vi "Product Page.vi"() -> (0 "Error Out":errorcluster)   [LabVIEW 2013, in "LVH-XBMC.lvlib"]
uses:
  vi.lib/LabVIEW Hacker/XBMC/LVH-XBMC.lvlib
  <vilib>/Platform/browser.llb/Open URL in Default Browser (string).vi
  <vilib>/LabVIEW Hacker/LVH-Toolbox/Common/LVH-Common.lvlib
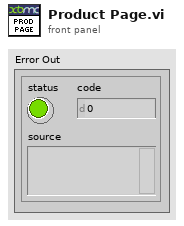
[diagram p1: front panel]
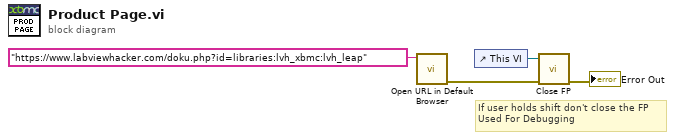
[diagram p0: block diagram]
diagram:
  # "If user holds shift don't close the FP\nUsed For Debugging"
  n1 = call-poly <vilib>:"Open URL in Default Browser.vi"("URL"="https://www.labviewhacker.com/doku.php?id=libraries:lvh_xbmc:lvh_leap") -> ("error out"=w1:errorcluster)  [unwired: 5 in, 1 out]
  n2 = control-ref of="This VI"() -> (w2:refnum<vi>)
  n3 = call <vilib>:"Close FP.vi"("Error In"=w1, "VI Ref"=w2) -> ("Error Out"=→"Error Out":errorcluster)  [unwired: 9 in]
